vi "Post Process Count Convert.vi"(0 "pInputImage":i32, 1 "pOutputImage":i32, 2 "iOutputBufferSize":i32, 3 "iNumImages":i32, 4 "iBaseline":i32, 5 "iMode":i32, 6 "iEmGain":i32, 7 "error in (no error)":errorcluster, 8 "fQE":sgl, 9 "fSensitivity":sgl, 10 "iHeight":i32, 11 "iWidth":i32) -> (20 "pInputImage out":i32, 21 "pOutputImage out":i32, 22 "function return":u32, 27 "error out":errorcluster)   [LabVIEW 2014, in "atmcd32d.lvlib"]
doc: "unsigned int WINAPI PostProcessCountConvert(at_32 * pInputImage, at_32 * pOutputImage, int iOutputBufferSize, int iNumImages, int iBaseline, int iMode, int iEmGain, float fQE, float fSensitivity, int iHeight, int iWidth);"
uses:
  atmcd32d.lvlib
  atmcd32d.dll
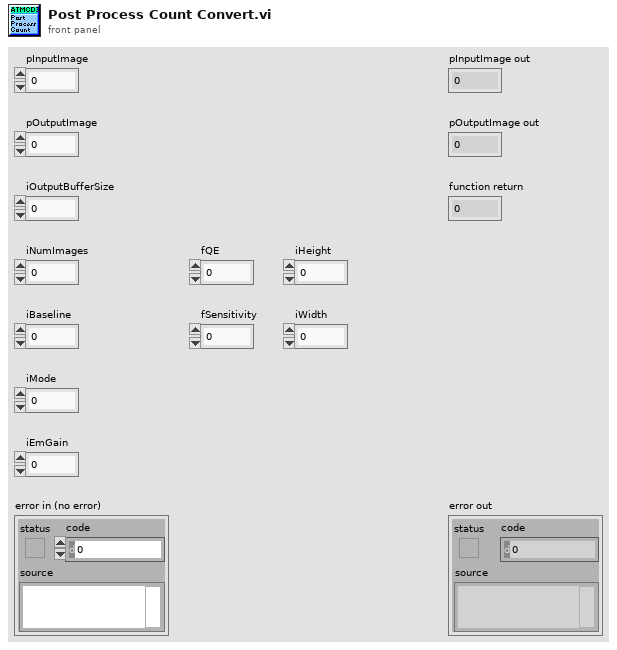
[diagram p1: front panel]
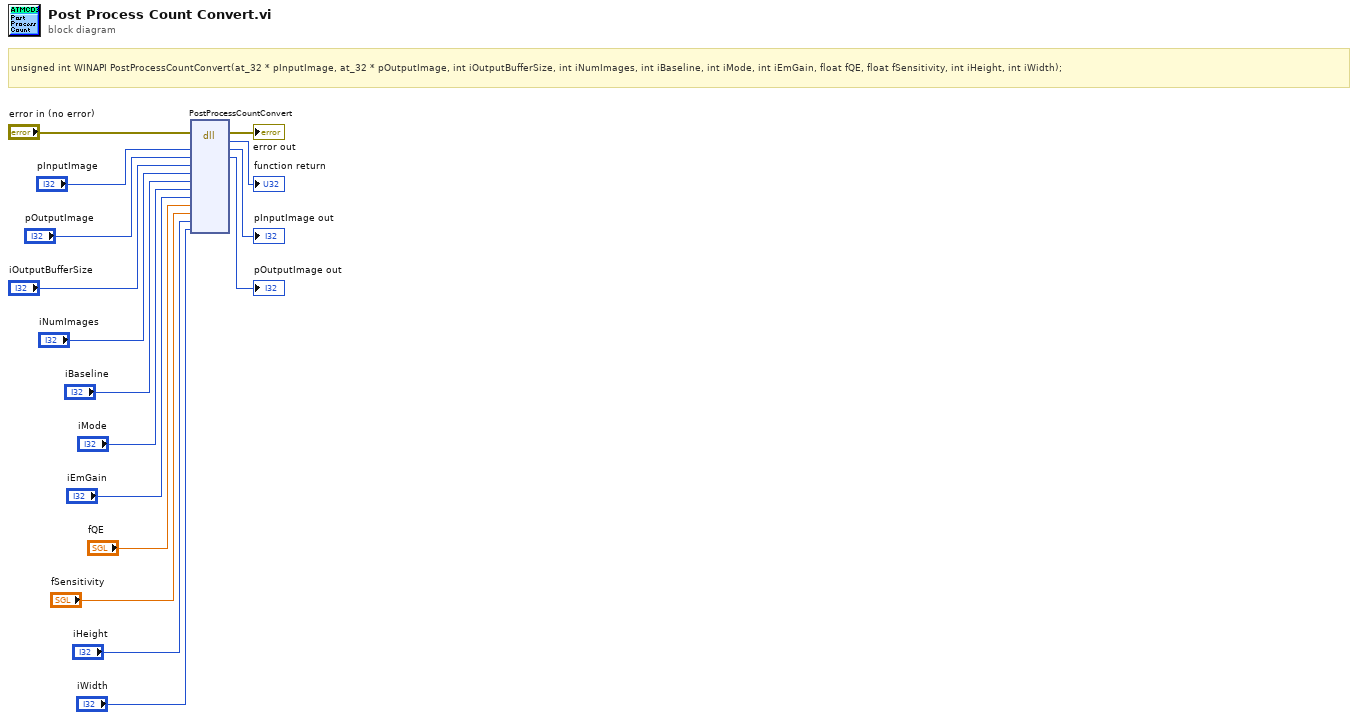
[diagram p0: block diagram]
diagram:
  # "unsigned int WINAPI PostProcessCountConvert(at_32 * pInputImage, at_32 * pOutputImage, int iOutputBufferSize, int iNumImages, int iBaseline, int iMode, int iEmGain, float fQE, float fSensitivity, int iHeight, int iWidth);"
  n1 = dll-call lib="C:/Users/Bakir/Documents/Lambda2-Testing/lib/Andorlib/atmcd32d.*" fn="PostProcessCountConvert"(error in="error in (no error)", "pInputImage"="pInputImage", "pOutputImage"="pOutputImage", "iOutputBufferSize"="iOutputBufferSize", "iNumImages"="iNumImages", "iBaseline"="iBaseline", "iMode"="iMode", "iEmGain"="iEmGain", "fQE"="fQE", "fSensitivity"="fSensitivity", "iHeight"="iHeight", "iWidth"="iWidth") -> (error out=→"error out":errorcluster, →"function return":u32, "pInputImage"=→"pInputImage out":i32, "pOutputImage"=→"pOutputImage out":i32)  [unwired: 11 in, 1 out]
